vi "Test Error.vi"   [LabVIEW 2020, in "Caraya Test 4.lvlib"]
uses:
  Caraya Test 4.lvlib
  <vilib>/addons/_JKI Toolkits/Caraya/classes/Assert/Assert Error.vi
  <vilib>/addons/_JKI Toolkits/Caraya/classes/Test/Test.lvclass
  <vilib>/addons/_JKI Toolkits/Caraya/classes/Assert/Assert.lvclass
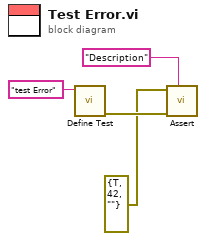
[diagram p0: block diagram]
diagram:
  n1 = call <vilib>:"Define Test.vi"("Label (VI Title)"="test Error" ("Description")) -> ("error out"=w4:errorcluster)  [unwired: 10 in]
  n2 = call-poly <vilib>:"Assert.vi"("Label"="Description" ("Description"), "error in (no error)"=w4, "Error?"=errorcluster {"status"=TRUE, "code"=42, "source"=""} ("error in (no error)")) -> ()  [unwired: 8 in, 1 out]
